vi "test_buffer_2.vi"() -> ()   [LabVIEW 2018]
uses:
  <vilib>/Instr/_visa.llb/VISA Configure Serial Port (Instr).vi
  <vilib>/Utility/file.llb/Write Delimited Spreadsheet (I64).vi
panel:
  in  "저장경로":path
  out "Estop?":bool
  out "숫자":i16
  out "(hi.lo)":i64=-193
  out "Upper to PCU":string
  in  "VISA resource name 2":refnum<visa-resource-name>="PCU"
  out "message":string="에러 없음" caption="메시지"
  out "PCU to Upper":string
  out "엔코더부터 끝까지 문자열":string="?ÿÿÿ"
  out "Gear(FB)":u8=2
  out "Speed0(FB)":u8
  out "Speed1(FB)":u8
  out "Steer0(FB)":u8=5
  out "Steer1(FB)":u8=1
  out "Brake(FB)":u8=1
  out "부호없는 바이트 배열":u8[](array[numeric])=[2, 0, 0, 5, 1, 1, 63, 255, 255, 255]
  out "잘라낸 STX":string="STX"
  out "잘라낸 EXT0과 1":string="\r\n"
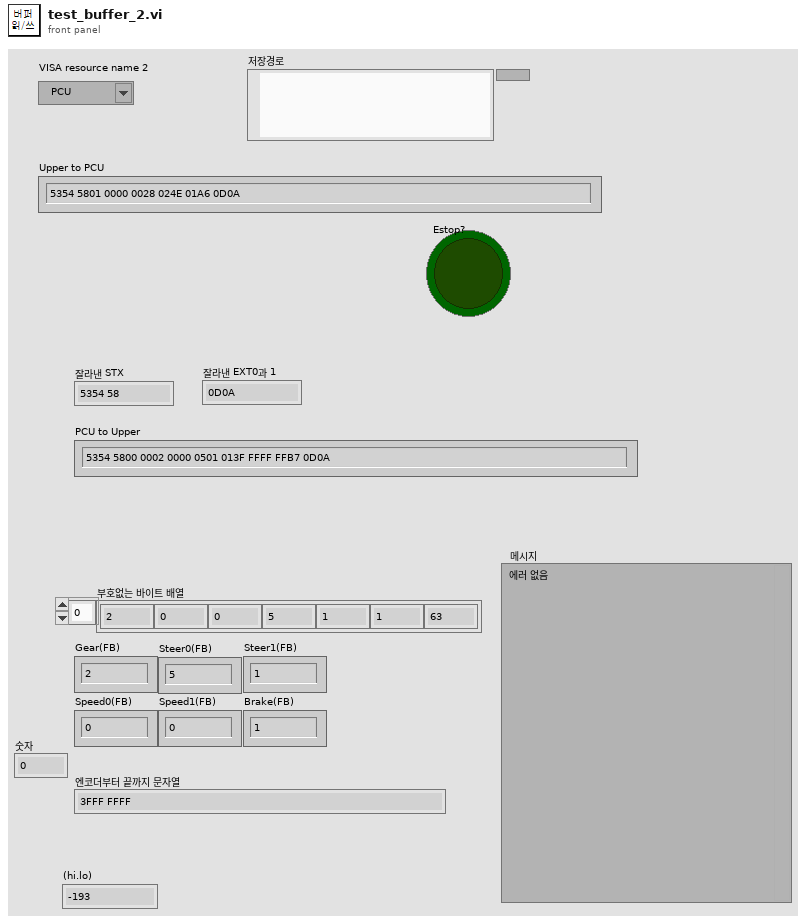
[diagram p1: front panel]
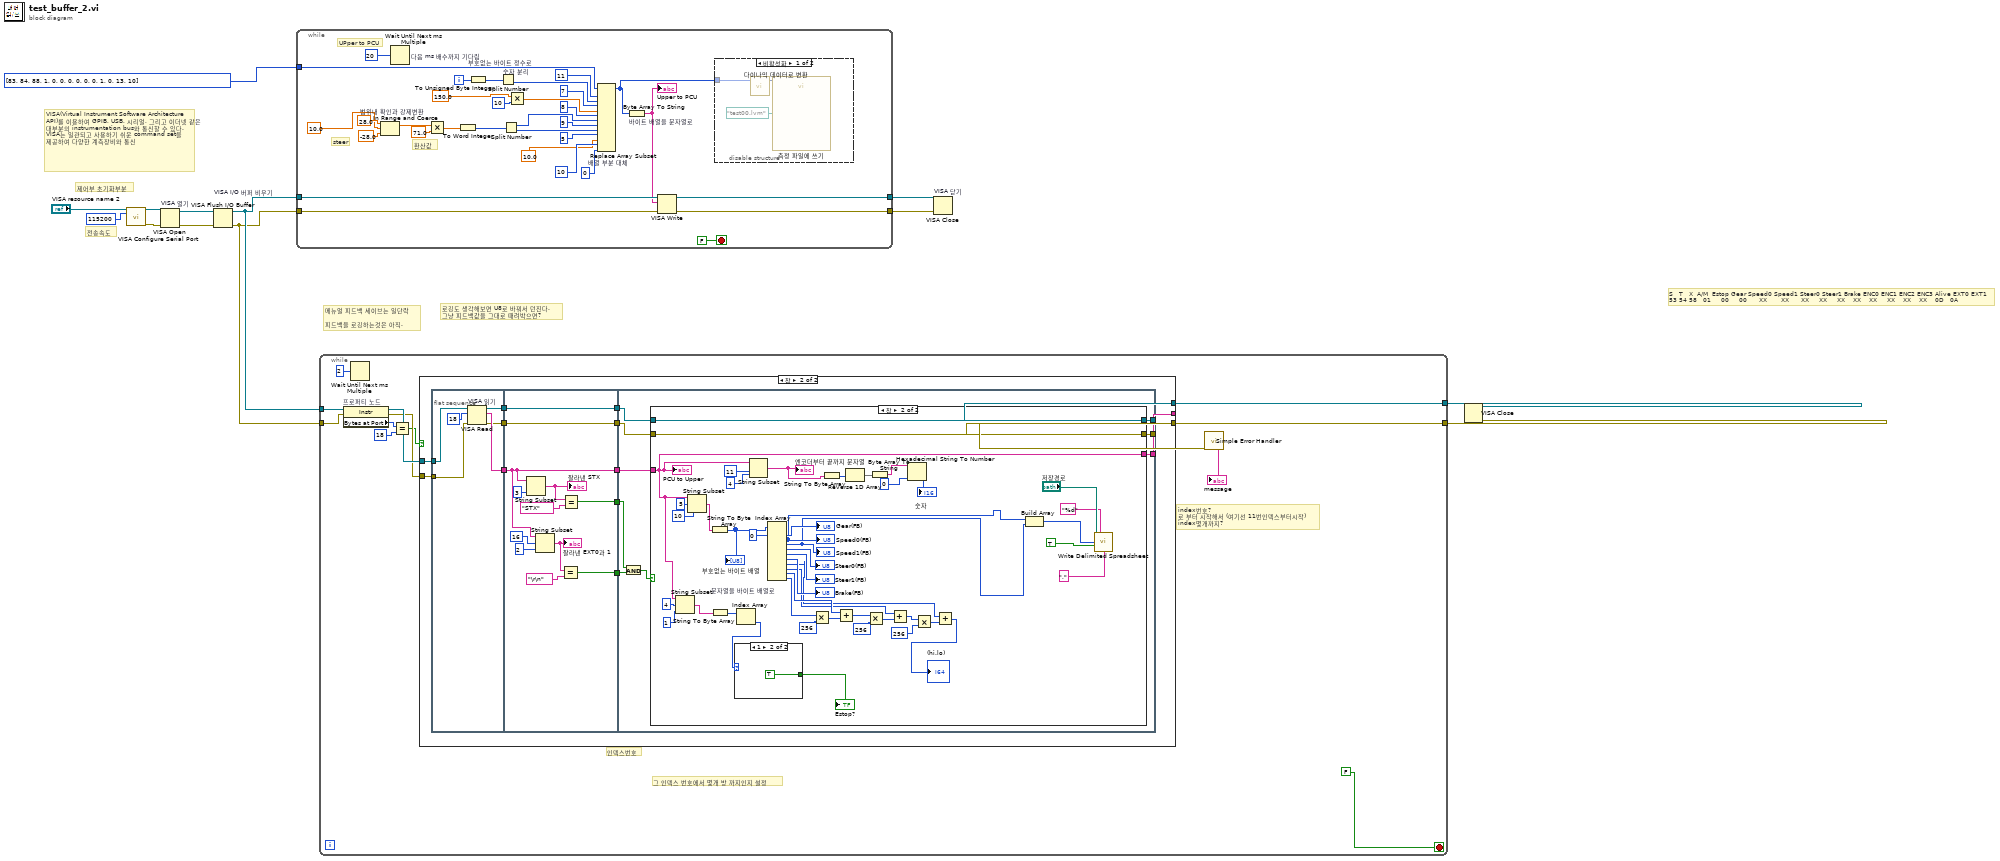
[diagram p0: block diagram]
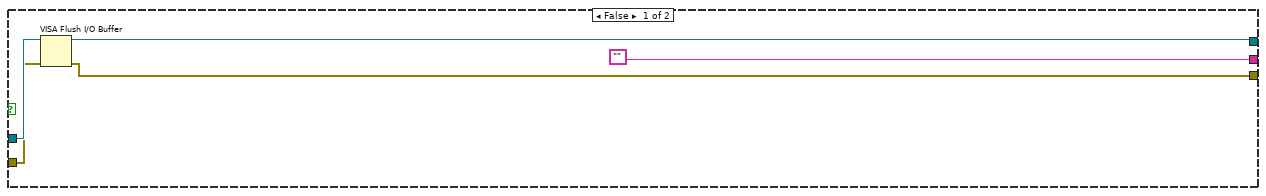
[diagram p3: hidden frame]
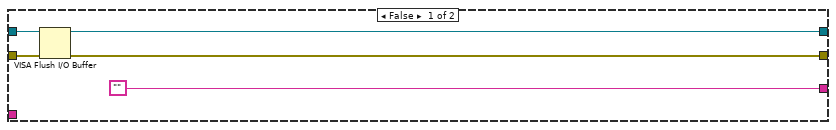
[diagram p4: hidden frame]
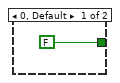
[diagram p5: hidden frame]
diagram:
  # "전송속도"
  # "VISA(Virtual Instrument Software Architecture API)를 이용하여 GPIB, USB, 시리얼, 그리고 이더넷 같은 대부분의 instrumentation bus와 통신할 수 있다. VISA는 일관되고 사용하기 쉬운 command set을 제공하여 다양한 계측장비와 통신"
  # "제어부 초기화부분"
  # "로깅도 생각해보면 U8로 바꿔서 던진다.\n그냥 피드백값을 그대로 때려박으면?"
  # "메뉴얼 피드백 세이브는 일단락\n\n피드백을 로깅하는것은 아직."
  # "S   T   X  A/M  Estop Gear Speed0 Speed1 Steer0 Steer1 Brake ENC0 ENC1 ENC2 ENC3 Alive EXT0 EXT1\n53 54 58   01     00     00      XX       XX      XX     XX     XX    XX    XX     XX    XX    XX    0D   0A"
  n1 = call-poly "VISA Configure Serial Port"("VISA resource name"="VISA resource name 2", "baud rate (9600)"=u32 115200) -> ("VISA resource name out"=w5:refnum<visa-resource-name>, "error out"=w6:errorcluster)  [unwired: 12 in]
  n2 = VISA Open "VISA 열기"(error in (no error)=w6, VISA resource name=w5) -> (VISA resource name=w4:refnum<visa-resource-name>, error out=w3:errorcluster)  [unwired: 3 in]
  n3 = VISA Flush I/O Buffer "VISA I/O 버퍼 비우기"(VISA resource name=w4, error in (no error)=w3) -> (VISA resource name out=w2:refnum<visa-resource-name>, error out=w1:errorcluster)  [unwired: 1 in]
  n4 = while {
    tunnel: w2 -> [w45]
    tunnel: w1 -> [w27]
    tunnel: [w44] -> w7
    tunnel: [w43] -> w8
    tunnel: u8[] [83, 84, 88, 1, 0, 0, 0, 0, 0, 0, 1, 0, 13, 10] ("기본값") -> [w41]
    i -> [w40]
    stop <- FALSE stop-if-true
    # "steer"
    # "환산값"
    # "UPper to PCU"
    n5 = In Range and Coerce "범위내 확인과 강제변환"(upper limit=28.0 ("상위 리미트"), x=10.0, lower limit=-28.0 ("하위 리미트")) -> (coerced(x)=w22:dbl)  [unwired: 1 out]
    n6 = Wait Until Next ms Multiple "다음 ms 배수까지 기다림"(millisecond multiple=u32 20) -> ()  [unwired: 1 out]
    n7 = Multiply(x=w22, y=71.0) -> (x*y=w24:dbl)
    n8 = To Word Integer(number=w24) -> (16bit integer=w23:i16)
    n9 = To Unsigned Byte Integer "부호없는 바이트 정수로"(number=w40) -> (unsigned 8bit integer=w38:u8)
    n10 = Split Number "숫자 분리"(x=w38) -> (lo(x)=w37:u8)  [unwired: 1 out]
    n11 = Split Number(x=w23) -> (hi(x)=w30:u8, lo(x)=w29:u8)
    n12 = Multiply(x=150.0, y=u8 10) -> (x*y=w34:dbl)
    n13 = Replace Array Subset "배열 부분 대체"(array=w41, new element #1=w37, index #1=11 ("인덱스"), new element #2=w34, index #2=7 ("인덱스"), new element #3=w30, index #3=8 ("인덱스"), new element #4=w29, index #4=9 ("인덱스"), new element #5=10.0, index #5=5 ("인덱스"), new element #6=u8 0 ("새 원소/부분배열"), index #6=10 ("인덱스")) -> (w14:u8[])
    n14 = Byte Array To String "바이트 배열을 문자열로"(unsigned byte array=w14) -> (string=w28:string)
    "Upper to PCU" <- w28
    n15 = VISA Write(VISA resource name=w45, write buffer=w28, error in (no error)=w27) -> (VISA resource name out=w44:refnum<visa-resource-name>, error out=w43:errorcluster)  [unwired: 1 out]
    n16 = disable-structure shown="비활성화" {
      disable-tunnel: w14 -> [w48 _]
      frame Disabled {
        n17 = call "다이나믹 데이터로 변환"("Array"=w48) -> ("Dynamic Data Type"=w47:dynamicdata)  [unwired: 3 in]
        n18 = call "측정 파일에 쓰기"("Signals"=w47, "Filename"=path "test00.lvm") -> ()  [unwired: 15 in, 3 out]
      }
      frame Enabled {
      }
    }
  }
  n19 = while {
    tunnel: w2 -> [w59]
    tunnel: w1 -> [w55]
    tunnel: [w51] -> w13
    tunnel: [w50] -> w12
    stop <- FALSE stop-if-true
    # "인덱스번호"
    # "그 인덱스 번호에서 몇개 방 까지인지 설정"
    # "index번호?\n로 부터 시작해서 (여기선 11번인덱스부터시작)\nindex몇개까지?"
    n20 = property on="프로퍼티 노드" class="Instr"(reference=w59, error in=w55) -> (reference out=w58:refnum<visa-resource-name>, error out=w57:errorcluster, "Bytes at Port"=w54:u32)
    n21 = Wait Until Next ms Multiple(millisecond multiple=u32 2) -> ()  [unwired: 1 out]
    n22 = Equal?(x=w54, y=u32 18) -> (x = y?=w52:bool)
    n23 = case shown="참" w52 {
      tunnel: w58 -> [w64 w78]
      tunnel: w57 -> [w63 w77]
      tunnel: ["" w66] -> _
      tunnel: [w62 w67] -> w50
      tunnel: [w61 w68] -> w51
      frame False {
        n24 = VISA Flush I/O Buffer(VISA resource name=w64, error in (no error)=w63) -> (VISA resource name out=w61:refnum<visa-resource-name>, error out=w62:errorcluster)  [unwired: 1 in]
      }
      frame True {
        n25 = flat-sequence {
          tunnel: w78 -> [w83]
          tunnel: w77 -> [w82]
          tunnel: [w81] -> w76
          tunnel: [w80] -> w71
          tunnel: [w79] -> w69
          tunnel: w76 -> [w87]
          tunnel: [w89] -> w75
          tunnel: [w88] -> w74
          tunnel: [w87] -> w73
          tunnel: [w86] -> w72
          tunnel: w71 -> [w86]
          tunnel: [w85] -> w70
          tunnel: w69 -> [w85]
          tunnel: w75 -> [w104]
          tunnel: w74 -> [w103]
          tunnel: w73 -> [w102]
          tunnel: w72 -> [w101]
          tunnel: w70 -> [w100]
          tunnel: [w99] -> w68
          tunnel: [w98] -> w67
          tunnel: [w97] -> w66
          frame #0 {
            n26 = VISA Read "VISA 읽기"(VISA resource name=w83, byte count=u32 18 ("바이트 카운트"), error in (no error)=w82) -> (VISA resource name out=w80:refnum<visa-resource-name>, read buffer=w81:string, error out=w79:errorcluster)  [unwired: 1 out]
          }
          frame #1 {
            n27 = String Subset(string=w87, length (rest)=3 ("길이(나머지)")) -> (substring=w95:string)  [unwired: 1 in]
            "잘라낸 STX" <- w95
            n28 = String Subset(string=w87, offset (0)=16 ("오프셋(0)"), length (rest)=2 ("길이(나머지)")) -> (substring=w93:string)
            "잘라낸 EXT0과 1" <- w93
            n29 = Equal?(x=w93, y="\r\n") -> (x = y?=w89:bool)
            n30 = Equal?(x=w95, y="STX") -> (x = y?=w88:bool)
          }
          frame #2 {
            n31 = And(x=w103, y=w104) -> (x .and. y?=w105:bool)
            n32 = case shown="참" w105 {
              tunnel: w102 -> [_ w123]
              tunnel: w101 -> [w110 w156]
              tunnel: w100 -> [w109 w118]
              tunnel: [w108 w156] -> w99
              tunnel: [w107 w118] -> w98
              tunnel: ["" w123] -> w97
              frame False {
                n33 = VISA Flush I/O Buffer(VISA resource name=w110, error in (no error)=w109) -> (VISA resource name out=w108:refnum<visa-resource-name>, error out=w107:errorcluster)  [unwired: 1 in]
              }
              frame True {
                n34 = String Subset(string=w123, offset (0)=4 ("오프셋(0)"), length (rest)=1 ("길이(나머지)")) -> (substring=w122:string)
                n35 = String Subset(string=w123, offset (0)=5 ("오프셋(0)"), length (rest)=10 ("길이(나머지)")) -> (substring=w150:string)
                n36 = String To Byte Array(string=w150) -> (unsigned byte array=w151:u8[])
                "부호없는 바이트 배열" <- w151
                n37 = String To Byte Array "문자열을 바이트 배열로"(string=w122) -> (unsigned byte array=w121:u8[])
                n38 = Index Array(array=w121) -> (element=w120:u8)  [unwired: 1 in]
                n39 = case shown="1" w120 {
                  tunnel: [FALSE TRUE] -> w119
                  frame 0, Default {
                  }
                  frame 1 {
                  }
                }
                "Estop?" <- w119
                n40 = String Subset(string=w123, offset (0)=u32 11 ("초기 스캔 위치"), length (rest)=4 ("길이(나머지)")) -> (substring=w144:string)
                "엔코더부터 끝까지 문자열" <- w144
                n41 = Index Array(array=w151, index #1=0 ("인덱스")) -> (element #1=→"Gear(FB)":u8, element #2=w117:u8, element #3=w116:u8, element #4=→"Steer0(FB)":u8, element #5=→"Steer1(FB)":u8, element #6=→"Brake(FB)":u8, element #7=w127:u8, element #8=w131:u8, element #9=w135:u8, element #10=w137:u8)  [unwired: 9 in]
                "Speed0(FB)" <- w117
                "Speed1(FB)" <- w116
                n42 = Multiply(x=w137, y=i16 256) -> (x*y=w136:i16)
                n43 = String To Byte Array(string=w144) -> (unsigned byte array=w143:u8[])
                n44 = Add(x=w135, y=w136) -> (x+y=w132:i16)
                n45 = Reverse 1D Array(array=w143) -> (reversed array=w142:u8[])
                n46 = Multiply(x=w132, y=i16 256) -> (x*y=w134:i16)
                n47 = Byte Array To String(unsigned byte array=w142) -> (string=w141:string)
                n48 = Add(x=w131, y=w134) -> (x+y=w128:i16)
                n49 = Hexadecimal String To Number(string=w141, default (0uL)=i16 0 ("기본(0 U32)")) -> (number=→"숫자":i16)  [unwired: 1 in, 1 out]
                n50 = Multiply(x=w128, y=i16 256) -> (x*y=w130:i16)
                n51 = Add(x=w127, y=w130) -> (x+y=→"(hi.lo)":i16)
                n52 = Build Array(w117, w116) -> (w115:u8[])
                n53 = call-poly <vilib>:"Write Delimited Spreadsheet.vi"("file path (dialog if empty)"="저장경로", "format (%d)"="%d" ("format (%s)"), "1D data"=w115, "append to file? (new file:F)"=TRUE, "delimiter (\\t)"="," ("delimiter (\\t)")) -> ()  [unwired: 9 in, 2 out]
                "PCU to Upper" <- w123
              }
            }
          }
        }
      }
    }
    n54 = call <vilib>:"Simple Error Handler.vi"("error in (no error)"=w50) -> ("message"=→"message":string)  [unwired: 4 in, 4 out]
  }
  n55 = VISA Close "VISA 닫기"(VISA resource name=w7, error in (no error)=w8) -> ()  [unwired: 1 out]
  n56 = VISA Close(VISA resource name=w13, error in (no error)=w12) -> ()  [unwired: 1 out]
